vi "Signal_generator.vi"() -> ()   [LabVIEW 2015]
panel:
  in  "IP address":string="161.111.10.5"
  in  "error in":errorcluster
  out "error out":errorcluster
  # "SIGNAL GENERATOR"
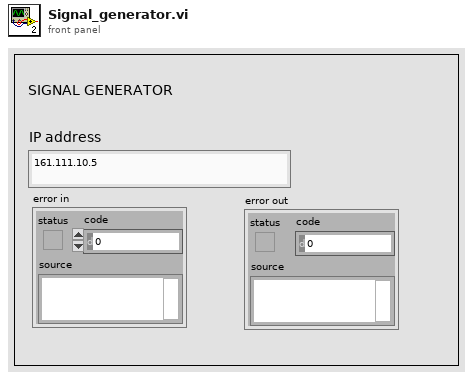
[diagram p1: front panel]
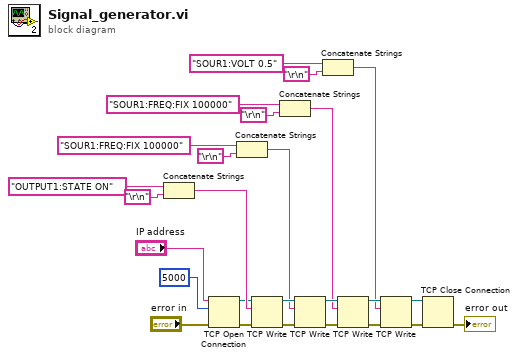
[diagram p0: block diagram]
diagram:
  n1 = Concatenate Strings("OUTPUT1:STATE ON" ("SCPI Message"), "\r\n") -> (w22:string)
  n2 = TCP Open Connection(address="IP address", remote port or service name=u16 5000, error in (no error)="error in") -> (connection ID=w20:refnum<k5>, error out=w19:errorcluster)  [unwired: 2 in]
  n3 = Concatenate Strings("SOUR1:FREQ:FIX 100000" ("SCPI Message"), "\r\n") -> (w5:string)
  n4 = TCP Write(connection ID=w20, data in=w22, error in (no error)=w19) -> (connection ID out=w17:refnum<k5>, error out=w16:errorcluster)  [unwired: 1 in, 1 out]
  n5 = Concatenate Strings("SOUR1:FREQ:FIX 100000" ("SCPI Message"), "\r\n") -> (w4:string)
  n6 = TCP Write(connection ID=w17, data in=w5, error in (no error)=w16) -> (connection ID out=w15:refnum<k5>, error out=w14:errorcluster)  [unwired: 1 in, 1 out]
  n7 = Concatenate Strings("SOUR1:VOLT 0.5" ("SCPI Message"), "\r\n") -> (w3:string)
  n8 = TCP Write(connection ID=w15, data in=w4, error in (no error)=w14) -> (connection ID out=w13:refnum<k5>, error out=w12:errorcluster)  [unwired: 1 in, 1 out]
  n9 = TCP Write(connection ID=w13, data in=w3, error in (no error)=w12) -> (connection ID out=w2:refnum<k5>, error out=w1:errorcluster)  [unwired: 1 in, 1 out]
  n10 = TCP Close Connection(connection ID=w2, error in (no error)=w1) -> (error out=→"error out":errorcluster)  [unwired: 1 in, 1 out]
